vi "AlliGator Phasor Harmonic Manager.vi"() -> ()   [LabVIEW 2021, in "AlliGator Phasor Harmonics.lvlib"]
uses:
  AlliGator Phasor Harmonics.lvlib
  Phasor/Phasor Harmonic Frequency Information.ctl
  Image/Image Control Refnum.ctl
  Globals, Variables, Constants/AlliGator Refnums List.ctl
  Phasor Plot/AlliGator Phasor Harmonic Manager Actions.ctl
  Image/Image Display Event.ctl
  <vilib>/Utility/miscctls.llb/LVPoint32TypeDef.ctl
  Globals, Variables, Constants/AlliGator Variables List.ctl
  Variant/Variant to Data/Variant to String.vi
  Globals, Variables, Constants/AlliGator Globals, Variables & Constants.lvlib
  Action Engine/AlliGator Action Engine.lvlib
  Notebook/Notebook.lvlib
  Notebook/AlliGator Notebook.lvlib
  Variant/Variant to Data/Variant to Data.lvlib
  Phasor Plot/AlliGator Phasor Plot.lvlib
  Image/Image.lvlib
  Rich Text Box/Rich Text Box.lvlib
  Phasor/Phasor.lvlib
panel:
  in  "Phasor Harmonic List":i32[](listbox) caption="ROI List"
  out "Dataset File Paths":path[](array[path])
  out "Phasor Harmonic Descriptions":string[](array[string])
  out "Harmonic Frequencies Information":T1[](array[typedef]) {"Base Frequency" format="%#_5g"; "Phasor Frequency" format="%#_5g"}
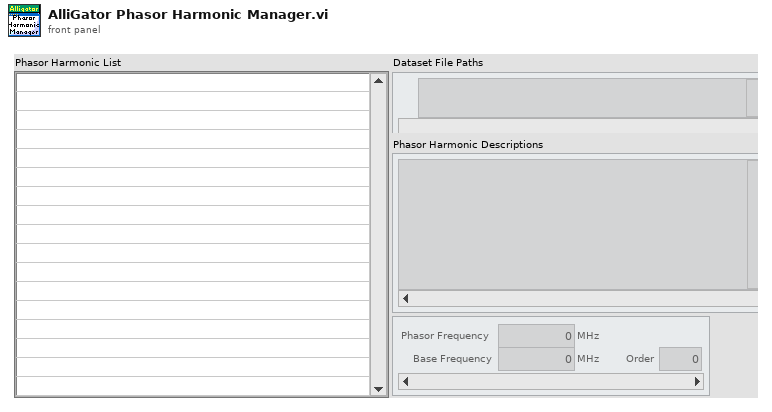
[diagram p1: front panel]
types:
  T1 = typedef "Phasor.lvlib/Phasor Harmonic Frequency Information.ctl" = cluster{"Phasor Frequency":dbl[unit], "Base Frequency":dbl[unit], "Order":u8}
  T2 = typedef "Image.lvlib/Image Control Refnum.ctl" = refnum<vi>
  T3 = typedef "AlliGator Globals, Variables & Constants.lvlib/AlliGator Refnums List.ctl" = enum16{"---------- AlliGator Controls ----------", "AlliGator Tab Control Refnum", "---------- AlliGator Indicators ----------", "Source Image Display Refnum", "Phasor Plot Display Refnum", "Decay Fit Parameter Map Refnum", "---------- AlliGator VIs ----------", "AlliGator Refnum", "AlliGator Settings Refnum", "AlliGator Launcher Refnum"}
  T4 = typedef "AlliGator Phasor Plot.lvlib/AlliGator Phasor Harmonic Manager Actions.ctl" = enum16{"Undefined", "Delete Current Harmonic", "Delete Multiple Harmonics", "Delete All Harmonics", "Swap Harmonics", "Insert Harmonics", "Rename Current Harmonic", "Store New Harmonic", "Store Multiple Harmonics", "Select Next Harmonic", "Select Previous Harmonic", "Update Phasor Harmonic Manager Window"}
  T5 = typedef "AlliGator Phasor Plot.lvlib/AlliGator Phasor Harmonic Manager Event Refnum.ctl" = refnum<user-event>
  T6 = typedef "Image.lvlib/Image Display Event.ctl" = cluster{"Item Tag":string, "Image Control Refnum":T2, "Coords":T7, "Item Path":string}
  T7 = typedef "LVPoint32TypeDef.ctl" = cluster{"Horizontal":i32, "Vertical":i32}
  T8 = typedef "AlliGator Globals, Variables & Constants.lvlib/AlliGator Variables List.ctl" = enum16{"---- GUI ----", "GUI:Initialization Status", "GUI:State Indicators Refnum", "GUI:Original AlliGator Menu Items", "GUI:Current Action Loop State", "GUI:Script in progress", "GUI:Playback", "GUI:Loop Playback", "GUI:Search ROI Used", "GUI:Search ROI", "Decay Graph Max Legend Size", "Intensity Graph Max Legend Size", "Decay Statistics Graph Max Legend Size", "Phasor Graph Max Legend Size", "Phasor Ratio Graph Max Legend Size", "Lifetime Graph Max Legend Size", "---- Files ----", "Files:Export Dataset Frames as Individual Files", "Files:Show Batch Export Help Balloons", "Files:Frames in Dataset", "Files:ptu File Frame Start Indices", "Files:Current Frame in Dataset", "Files:Current Frame Timestamp", "Files:Dataset Loaded", "Files:Dataset Metadata", "Files:Dataset Channel", "Files:Dataset Data Description", "Files:Background Dataset Metadata", "Files:Background Dataset Channel", "Files:Background Dataset Data Description", "Files:Background File Subtraction", "Files:Background File Path", "Files:Background File Pile-up Correction", "Files:Background File Pixel Well Capacity", "Files:Background File Scaling Factor", "Files:Current Dataset Load Settings", "Files:Dataset Path", "Files:ICCD-specific Information", "Files:Macrotime Gate Separation", "------ Python Plugins ------", "Python Plugins:Information", "Python Plugins:Python Session", "Python Plugins:Valid Python Session?", "---- Source Image ----", "Source Image:ROIs", "Source Image:Current ROI", "Source Image:ROI Event Refnum", "X_Source Image:Display Range", "X_Source Image:Palette Information", "X_Source Image:Type of Displayed Image", "X_Time Gate Slider", "Source Image:Palette List", "Source Image:Scale", "Source Image:ROI Overlay Color", "Source Image:Overlay to Erase", "Source Image:Is Displayed Image Accumulated", "Source Image:White Light Image Modified", "Source Image:Mask Image Modified", "---- Image Profile Window ----", "Image Profile:Window Event Refnum", "Image Profile:IntensityType", "Image Profile:Intensity Average Type", "Image Profile:Intensity-weighted SDV", "Image Profile:Box Profile Type", "Image Profile:Window Open", "Image Profile:Plotted Fit Parameter", "------ Phasor Graph -------", "Phasor Graph:Show Line", "---- Phasor Plot ---", "Phasor Plot:Parameters Changed", "Phasor Plot:FLI Dataset Modified since last Calculation", "Phasor Harmonics Data", "Selected Phasor Harmonics", "Phasor Harmonic Manager Event Refnum", "Phasor Plot:ROIs", "Phasor Plot:Current ROI", "Phasor Plot:ROI Event Refnum", "Phasor Plot:Image Reference Points", "Phasor Plot:Computed", "Phasor Plot:Palette Information", "Phasor Plot:Palette List", "Phasor Plot:Phasor Ratio Palette Information", "Phasor Plot:Phasor Ratio Palette List", "Phasor Plot:Image Scale", "Phasor Plot:Image Overlay to Erase", "Phasor Plot:Image Elements to Update", "Phasor Plot:Current Calculation Parameters", "Phasor Plot:Current Calibration Options", "Phasor Plot:Reset Cumulated Phasor Plot", "Phasor Plot:Reference 1", "Phasor Plot:Lifetime Reference 1", "Phasor Plot:Reference 1 Frequency", "Phasor Plot:Reference 2", "Phasor Plot:Lifetime Reference 2", "Phasor Plot:Reference 2 Frequency", "---- Decay Analysis ----", "Number of Selected Decays to Fit", "LS Fit Results", "LAR Fit Results", "BS Fit Results", "Last Decay Max - Min", "Best Fit Parameters", "Best Fit Parameter Names", "Actual Size X", "Actual Size Y", "Binning X", "Binning Y", "Actual # Gates", "Dataset Number", "Gates to...", "Gates Skipped", "Gates to keep", "Gate Step", "Gate Separation", "Reversed Gates", "Pile-up Correction", "Pixel Well Capacity", "Background Subtracted", "Background Subtraction Method", "Background Definition Range", "Background File (deprecated)", "Number of Dataset Accumulated", "Array of Accumulated Dataset Paths", "Do Averaged Datasets", "Destination File Path", "Process Plot Target", "Use 1/D as Phasor Frequency", "---- Decay Fit Parameter Map -----", "Decay Fit Parameter Map:Palette Information", "Decay Fit Parameter Map:Palette List", "Decay Fit Parameter Map:X Resolution", "Decay Fit Parameter Map:Y Resolution", "---- Parameter Map ----", "Parameter Map:Palette Information", "Parameter Map:Palette List", "------- Local Decay Window ---------", "Local Decay Graph Window:Event Refnum", "Local Decay Graph Window:Use normalized IRF for convolution", "----- Miscellaneous ----", "Misc:Skippable Dialog Windows Status"}
  T9 = cluster{"data name":string, "drag data":variant}[]
  T10 = typedef "AlliGator Action Engine.lvlib/AlliGator Q Element.ctl" = cluster{"AlliGator Q Event":T11, "Data":variant}
  T11 = typedef "AlliGator Action Engine.lvlib/AlliGator Q Event.ctl" = enum16{"---- Files ----", "Files:Set Batch Export Files To Save", "Files:Set Dataset Loading & Pre-processing Options", "Files:Check #Frames in Dataset", "Files:Increment Frame Index", "Files:Open Mask Image", "Files:Open White Light Image", "Files:Open Single Dataset", "Files:New Folder of Folders Selected", "Files:Load File (all Types)_Scriptable", "Files:Move Flattened Series to Folders Series", "Files:Select Folder", "Files:Load FLI Dataset", "Files:Load Swiss SPAD 1 Dataset", "Files:Load Swiss SPAD 2 Dataset", "Files:Load .sdt FLI Dataset", "Files:Load .ptu FLI Dataset", "Files:Load .bin FLI Dataset", "Files:Load Single Gate Image Folder", "Files:Load I/m/phi Dataset (deprecated)", "Files:Load Single Image", "Files:Subtract Background File", "Files:Export FLI Dataset", "Files:Load HDF5 FLI Dataset", "Files:Set Destination File Path", "Files:Save Mask Image", "Files:Batch Conversion", "Files:New Folder Selected", "Files:Close FLI Dataset", "Files:Close FLI Dataset Series", "Files:Close White Light Image", "Files:Close Mask Image", "---- FLI Dataset ----", "FLI Dataset:Channel Arithmetic", "FLI Dataset:Export Average Lifetime Map as ASCII", "FLI Dataset:Export User-Defined Quantity Map as ASCII", "FLI Dataset:Python Function FLI Dataset Event", "FLI Dataset:ROI Analysis", "FLI Dataset:Tilted Logistic Square Gated IRF Characteristics Map", "FLI Dataset:Logistic Square Gated IRF Characteristics Map", "FLI Dataset:Square Gated IRF Characteristics Map", "FLI Dataset:Multi-ROI Single-Pixel Phasor Analysis", "FLI Dataset:Multi-ROI Single-Pixel NLSF Analysis", "FLI Dataset:All ROIs IRF Extraction", "FLI Dataset:All ROIs Decay Fit Non-Interactive (Fast + Individual IRF)", "FLI Dataset:All ROIs Phasor Analysis", "FLI Dataset:All ROIs Decay Fit", "FLI Dataset:Fluorescence Decay Statistics", "FLI Dataset:Update Decay Statistics Graph", "FLI Dataset:Get Decay from ROI", "FLI Dataset:All ROIs Average Lifetimes", "FLI Dataset:Save/Load Local IRFs", "FLI Dataset:Clear Local IRFs", "---- FLI Dataset Series ----", "FLI Dataset Series:Sum All Datasets in Series", "FLI Dataset Series:Add Dataset to Accumulated Dataset", "FLI Dataset Series:Display Accumulated Dataset", "FLI Dataset Series:Clear Dataset Series Sum", "FLI Dataset Series:Time-Series Analysis (NLSF)", "FLI Dataset Series:Time-Series Analysis (Phasor)", "---- Image ----", "Image:Update Image Profile Plots", "Image:Image Histogram Cursor Move", "Image:Image Histogram", "Image:Image Contrast", "Image:Set Image Histogram Cursor Move Flag", "Image:Clear Image Overlay", "Image:Use ROI as Search Area", "Image:Set ROI Diameter", "Image:Save Image Data as TIFF", "Image:Save Displayed Image with Overlay", "Image:Save Image Overlay Only", "Image:Save Image as Hot Pixel Mask", "Image:Change Source Image Color Palette", "Image:Copy Image to Clipboard", "Image:Source Image ROI Selection", "Image:Delete All ROIs", "Image:Delete All Unselected ROIs", "Image:Delete ROI", "Image:Merge All ROIs", "Image:Store ROI", "Image:Source Image ROI Storage", "Image:Export ROI Description to Notebook", "Image:Save ROI", "Image:Load ROI", "Image:Paste ROI Definition", "Image:Clear ROI", "Image:Identify ROIs in Mask Image", "Image:Create Complementary ROI", "Image:Create Contour ROI", "Image:Create ROI(s) from Pixels with Peak above Min_Scriptable", "Image:Create ROI(s) from Pixels with Intensity above Min_Scriptable", "Image:Compute ROI Statistics", "Image:Delete ROI(s) based on ROI Characteristics", "Image:Create ROI Grid", "Image:ROI to Individual Pixel ROIs", "Image:Python Function Source Image Event", "Image:Show Phasor Calibration Map ROI Centers", "Image:Convert ROI to Mask Image", "Image:Mouse Move", "Image:Mouse Up", "Image:Set Source Image Mouse Move Flag", "Image:Add Scale Bar Overlay", "Image:Delete Existing ROIs Option", "Image:Overlay ROI Median", "Image:Check Current ROI", "---- Decay ----", "Decay:Clear IRF/Reference Plot", "Decay:Add Decay to Graph", "Decay:Smoothen Plot", "Decay:Smoothen Plot Tail", "Decay:Average Selected Plots", "Decay:Extract IRF", "Decay:Optimal IRF Extraction", "Decay:Threshold IRF", "Decay:Fit to Model IRF", "Decay:Fit IRF to Square Gate", "Decay:Fit IRF to Logistic Square Gate", "Decay:Fit IRF to Tilted Logistic Square Gate", "Decay:Create Bounding Cursors Set", "Decay:Export Bounding Cursors Definition to Notebook", "Decay:Denoise Plot", "Decay:Compute Cumulative Function", "Decay:Use as Reference Decay", "Decay:Show Reference Decay/IRF", "Decay:Extrapolate Decay", "Decay:Create Head & Tail Bounding Cursors", "Decay:Store Cursor-defined Head & Tail Fractions", "Decay:Rebin Plot", "Decay:1-Normalize Decay", "Decay:[0-1]-Normalize Plot", "Decay:Straighten Decay", "Decay:Shift Decay", "Decay:Fold Decay", "Decay:Fit Decay", "Decay:Global Fit of Selected Decays", "Decay:Post Global Fit Script", "Decay:Add Global Fit Parameters to Graph", "Decay:Add Decay Parameter(s) to Plot (Graph)", "Decay:Export Decay to Phasor Graph", "Decay:Plot Decay Shifts", "Decay:Compute Average Lifetime", "Decay:Plot Convolution", "Decay:Graph Tip Strip Update", "---- Decay Statistics ----", "Decay Statistics:Tip Strip Update", "---- Intensity Time Trace ----", "Intensity Time Trace:Use File Timestamp", "Intensity Time Trace:Load Intensity Corrections File", "Intensity Time Trace:Clear Intensity Corrections File", "Intensity Time Trace:Tip Strip Update", "---- Phasor Plot ----", "Phasor Plot:Build Phasor Plot", "Phasor Plot:Change Phasor Plot Color Palette", "Phasor Plot:Adjust Phasor Plot Display Range", "Phasor Plot:Highlight Image ROI in Phasor Plot", "Phasor Plot:Save Phasor Plot Image with Overlay", "Phasor Plot:Export Complex Phasor Map", "Phasor Plot:Export Phasor Ratio Map", "Phasor Plot:Export Average Lifetime Map", "Phasor Plot:Compute Phase Lifetime Histogram", "Phasor Plot:Compute Phasor Ratio Histogram", "Phasor Plot:Compute Phase Lifetime vs Intensity Scatter Plot", "Phasor Plot:Weber 2-Component Decomposition", "Phasor Plot:Update Phasor Color Map Vertices", "Phasor Plot:Clear Phasor Overlay", "Phasor Plot:Use Segment Extremities as References", "Phasor Plot:Use UC/Segment Intersections as References", "Phasor Plot:Use UC/Principal Axis Intersections as References", "Phasor Plot:Use UC/Linear Fit Intersections as References", "Phasor Plot:Update Phasor Plot Reference", "Phasor Plot:Show Local Phasor Info in Phasor Plot", "Phasor Plot:Update Phasor Plot State", "Phasor Plot:Phasor Plot ROI Storage", "Phasor Plot:Phasor Plot ROI Selection", "Phasor Plot:Python Function Phasor Plot Event", "Phasor Plot:Overlay Phasor ROI, Ratio or Map in Source Image", "Phasor Plot:Compute Decay of Selected Phasors", "Phasor Plot:Phasor at Image Pixel", "Phasor Plot:Mouse Move", "Phasor Plot:Mouse Up", "Phasor Plot:Display Range Mouse Move", "Phasor Plot:Set Mouse Move Flag", "---- Phasor Graph ----", "Phasor Graph:Calibrated Phasor Map Series", "Phasor Graph:Whole Image Phasor Scatter Plot (deprecated)", "Phasor Graph:Get Phasor Value", "Phasor Graph:Create New Phasor Plot Dialog", "Phasor Graph:Update Last Phasor Value", "Phasor Graph:Update Phasor (m, phi)", "Phasor Graph:Remove Single Phasor from Plot", "Phasor Graph:Add Single Phasor to Plot", "Phasor Graph:Remove Phasor Plot", "Phasor Graph:Remove Selected Phasor Plots", "Phasor Graph:Clear Phasor Data", "Phasor Graph:Clear Phasor Graph", "Phasor Graph:Cursor Move", "Phasor Graph:Draw Cursor Connecting Line", "Phasor Graph:Clear Cursor Connecting Line", "Phasor Graph:Find UC Intersection", "Phasor Graph:Use UC/Cursor-Defined Line Intersections", "Phasor Graph:Use Selected Plots Fitted Line/UC Intersections", "Phasor Graph:Use Selected Plots Principal Axis/UC Intersections", "Phasor Graph:Show Single Phasor", "Phasor Graph:Save Single Phasor Plot", "Phasor Graph:Save All Phasor Plots", "Phasor Graph:Load Phasor Plot(s)", "Phasor Graph:Phasor Multiplication", "Phasor Graph:Compute Average Phasor", "Phasor Graph:Compute Multiple Average Phasors (Selected Plots)", "Phasor Graph:Export Single Phasor Plot Phase Lifetimes", "Phasor Graph:Phase Lifetime Trajectory (deprecated)", "Phasor Graph:Phase Lifetime vs Intensity Scatter Plot (deprecated)", "Phasor Graph:Parameter 2 vs Parameter 1 Scatter Plot", "Phasor Graph:Use Cursor n Location", "Phasor Graph:Set Reference n to Current Phase Lifetime Value", "Phasor Graph:Set Reference n to Lifetime Value", "Phasor Graph:Set Cursor n Location", "Phasor Graph:Save Phasor Graph Image", "Phasor Graph:Update SEPL Plot", "Phasor Graph:Export Single Phasor Plot Data", "Phasor Graph:Export Selected Phasor Plots Data", "Phasor Graph:Python Function Phasor Graph Event", "Phasor Graph:Tip Strip Update", "---- Calibration ----", "Calibration:Set Calibration Type", "Calibration:Load/Save Phasor Calibration", "Calibration:Load/Save Phasor Calibration Series", "Calibration:Load/Save Phasor Calibration Map", "Calibration:Use as Calibration", "Calibration:Compute Optimal Calibration from Phasor References", "Calibration:Clear Phasor Calibration", "Calibration:Single Phasor Calibration Information", "Calibration:Use as Calibration Series", "Calibration:Use as Calibration Map", "Calibration:Clear Calibration Series", "Calibration:Phasor Calibration Series Information", "Calibration:Clear Calibration Map", "Calibration:Phasor Calibration Map Information", "Calibration:Apply Phasor Calibration", "Calibration:Update Single Plot Calibration", "Calibration:Update Multiple Plots Calibration", "Calibration:Clear Single Plot Calibration", "Calibration:Clear All Plots Calibrations", "Calibration:Clear Plot(s) Calibration(s)?", "Calibration:Phasor Calibration Maps (# Gates Series)", "---- Phasor Ratio ----", "Phasor Ratio:Clear Reference n", "Phasor Ratio:Toggle Selected Plot(s)  Lock to Reference 1", "Phasor Ratio:Use as Reference n", "Phasor Ratio:Send Reference n to Notebook", "Phasor Ratio:Toggle Selected Plot(s)  Lock to Reference 2", "Phasor Ratio:Compute Phasor Ratio at Mouse Location", "Phasor Ratio:Compute Phasor Plot's Average Phasor Ratio", "Phasor Ratio:Compute Time-Series Phasor Ratios", "Phasor Ratio:Fit Line to Phasor Ratio Plot", "Phasor Ratio:Save References", "Phasor Ratio:Load References", "Phasor Ratio:Update Phasor Reference 1", "Phasor Ratio:Update Phasor Reference 2", "Phasor Ratio:Move Cursor n to Reference n", "Phasor Ratio:Use as Phasor Reference 1 Lifetime", "Phasor Ratio:Use as Phasor Reference 2 Lifetime", "Phasor Ratio:Export Phasor Ratio Map as ASCII", "Phasor Ratio:Tip Strip Update", "---- Lifetime & Other Parameters Graph ----", "Lifetime:Power Law from Intensity Distribution", "---- Decay Fit Parameter Map ----", "Decay Fit Parameter Map:Export ROI NLSF Data as ASCII", "Decay Fit Parameter Map:Set Decay Fit Parameter Map Selection", "Decay Fit Parameter Map:Build Decay Fit Parameter Map", "Decay Fit Parameter Map:Change Decay Fit Parameter Map Color Palette", "Decay Fit Parameter Map:Export Decay Fit Parameter Map Data as ASCII", "Decay Fit Parameter Map:Export All Decay Fit Parameter Maps Data as ASCII", "Decay Fit Parameter Map:Selected Parameter Scatterplot", "Decay Fit Parameter Map:Parameter 2 vs Parameter 1 Scatterplot", "Decay Fit Parameter Map:Save Decay Fit Parameter Map Image", "Decay Fit Parameter Map:Save-Load IRFs & Fit Data", "Decay Fit Parameter Map:Update Local Decay Plots", "Decay Fit Parameter Map:Python Function Decay Fit Parameters Map Event", "Decay Fit Parameter Map:Overlay Decay Fit Parameter Map in Source Image", "Decay Fit Parameter Map:Selected Parameter vs Intensity Scatterplot", "Decay Fit Parameter Map:Mouse Up", "Decay Fit Parameter Map:Display Range Mouse Move", "Decay Fit Parameter Map:Change Map Resolution", "---- Parameter Map ----", "Parameter Map:Export ROI Parameters Data as ASCII", "Parameter Map:Delete Parameter Map Set", "Parameter Map:Update Parameter List", "Parameter Map:Build Parameter Map", "Parameter Map:Change Parameter Map Color Palette", "Parameter Map:Export Parameter Map Data as ASCII", "Parameter Map:Export All Parameter Maps Data as ASCII", "Parameter Map:Selected Parameter Scatterplot", "Parameter Map:Parameter 2 vs Parameter 1 Scatterplot", "Parameter Map:Selected Parameter vs Intensity Scatterplot", "Parameter Map:Save Parameter Map Image", "Parameter Map:Save-Load IRFs & Parameter Maps (TODO)", "Parameter Map:Set Parameter Map Selection", "Parameter Map:Python Function Parameter Map Event", "Parameter Map:Overlay Parameter Map in Source Image", "Parameter Map:Update Local Decay Plots", "Parameter Map:Mouse Up", "Parameter Map:Display Range Mouse Move", "---- Generic Graph ----", "Generic Graph:Generic XY Graph Event", "Generic Graph:Python Function XY Graph Event", "Generic Graph:New Plot", "Generic Graph:Save Plot", "Generic Graph:XY Plot Histogram", "Generic Graph:Set XY Graph Plot Name", "Generic Graph:Set Last Cursor Style", "Generic Graph:Tip Strip Update", "---- GUI ----", "GUI:Start Script", "GUI:Type of Displayed Image Changed", "GUI:Gate Image Slide Changed", "GUI:Show Busy Icon", "GUI:Show Busy Icon & Abort Button", "GUI:Hide Busy Icon", "GUI:Hide Busy Icon & Abort Button", "GUI:Abort", "GUI:End Script", "GUI:Start Timing", "GUI:End Timing", "GUI:Set State Indicator", "GUI:Send Parameters JSON Strings to Clipboard", "GUI:Set Gate Step", "GUI:Idle", "GUI:Initialization", "GUI:Quit", "GUI:Increment Dataset Index", "GUI:Set Dataset Index to -1", "GUI:Time Series Slider Moved", "GUI:Time Series Slider Changed", "GUI:Toggle Playback or Loop", "GUI:Playback Script", "GUI:Set Phasor Frequency", "GUI:Open Window", "GUI:Start Test Script", "GUI:End Test Script", "DEBUG"}
  T12 = typedef "Rich Text Box.lvlib/Text Formatting.ctl" = cluster{"Font":string, "Text Color":T13, "Text Background Color":T13, "Text Style":enum16{"Regular", "Bold", "Italic", "Underline", "Strikeout"}, "Font Size (Points)":dbl, "Text Alignment":i32}
  T13 = typedef "Rich Text Box.lvlib/Text Colors.ctl" = enum16{"Unchanged", "Black", "Blue", "Brown", "Gray", "Green", "Orange", "Pink", "Red", "White"}
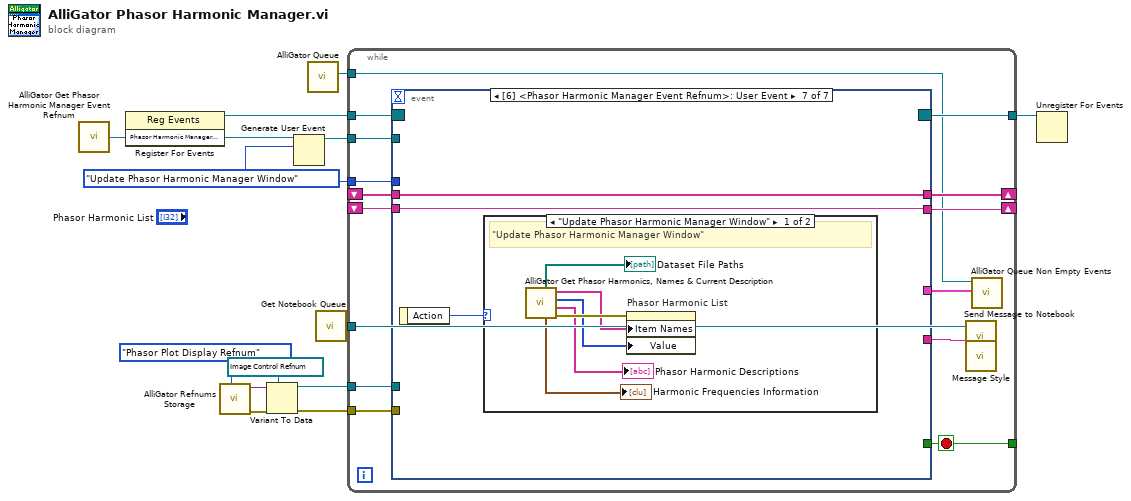
[diagram p0: block diagram]
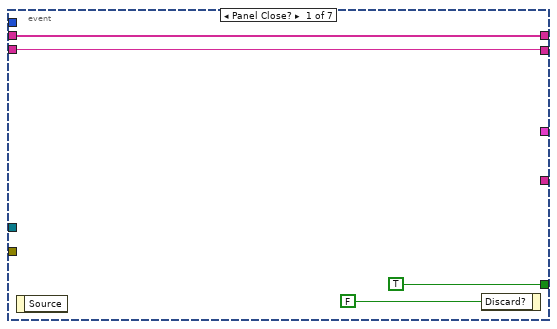
[diagram p2: hidden frame]
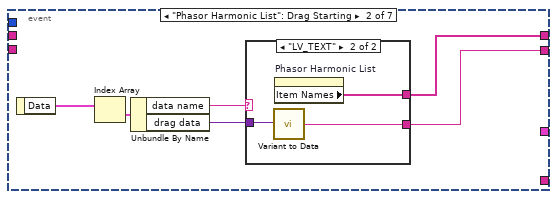
[diagram p3: hidden frame]
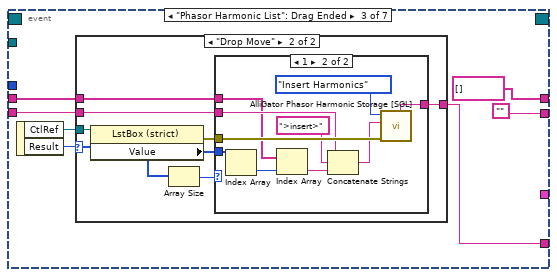
[diagram p5: hidden frame]
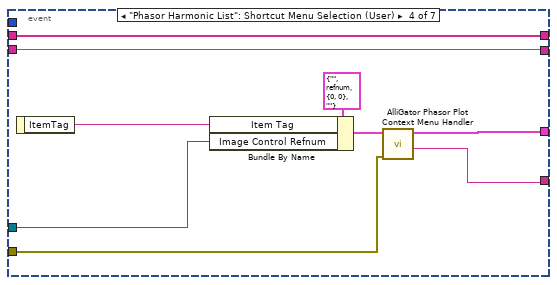
[diagram p8: hidden frame]
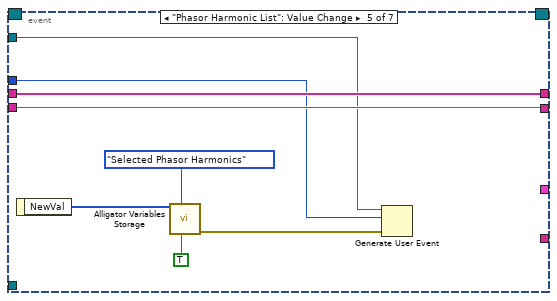
[diagram p9: hidden frame]
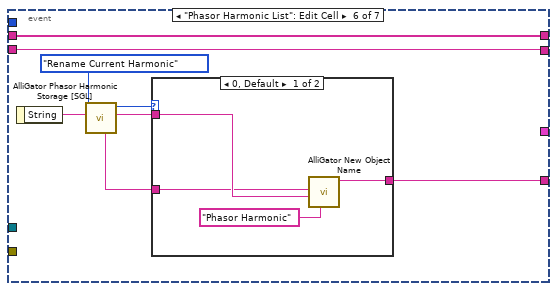
[diagram p10: hidden frame]
diagram:
  w7 = AlliGator_Phasor_Harmonic_Manager_Actions."Update Phasor Harmonic Manager Window" ("event data")
  n1 = call "AlliGator Get Phasor Harmonic Manager Event Refnum.vi"() -> ("Phasor Harmonic Manager Event Refnum"=w9:T5)
  n2 = register-events(w9) -> (reference out=w13:refnum<event-registration>)  [unwired: 2 in, 1 out]
  n3 = call "AlliGator Refnums Storage.vi"("AlliGator Refnum List"=AlliGator_Refnums_List."Phasor Plot Display Refnum") -> ("Error Out"=w6:errorcluster, "Data out"=w5:variant)  [unwired: 9 in]
  n4 = Variant To Data(error in=w6, type=T2 refnum ("Image Control Refnum"), Variant=w5) -> (data=w1:T2, error out=w3:errorcluster)
  n5 = Generate User Event(user event=w9, event data cluster=w7) -> (user event out=w8:T5)  [unwired: 2 in, 1 out]
  n6 = call "AlliGator Queue.vi"() -> ("AlliGator Q"=w11:refnum<queue>)  [unwired: 8 in, 1 out]
  n7 = call "Get Notebook Queue.vi"() -> ("Notebook Queue"=w10:refnum<queue>)  [unwired: 9 in]
  n8 = while {
    tunnel: w13 -> [w29]
    tunnel: [w28] -> w12
    tunnel: w11 -> [w20]
    tunnel: w10 -> [w14]
    shift-right: [w27] -> _
    shift-left: _ -> [w26]
    shift-right: [w25] -> _
    shift-left: _ -> [w24]
    tunnel: w8 -> [w23]
    tunnel: w7 -> [w22]
    tunnel: [w21] -> _
    tunnel: w3 -> [w18]
    tunnel: w1 -> [w17]
    stop <- w21 stop-if-true
    n9 = event shown="[6] <Phasor Harmonic Manager Event Refnum>: User Event" {
      selector: w29 -> [_ _ _ _ _ _ _]
      dyn-events: [_ _ _ _ _ _ _] -> w28
      timeout: _ -> [_ _ _ _ _ _ _]
      tunnel: [TRUE _ _ _ _ _ _] -> w21
      tunnel: [w31 w36 "" w75 w82 w91 w98] -> w27
      tunnel: w26 -> [w31 _ w47 w75 w82 w91 w98]
      tunnel: [w30 w34 string[] [] ("Item Names") w74 w81 w90 w97] -> w25
      tunnel: w24 -> [w30 _ w45 w74 w81 w90 w97]
      tunnel: w23 -> [_ _ _ _ w78 _ _]
      tunnel: w22 -> [_ _ _ _ w77 _ _]
      tunnel: [_ _ _ w71 _ _ _] -> w19
      tunnel: w18 -> [_ _ _ w69 _ _ _]
      tunnel: w17 -> [_ _ _ w68 _ _ _]
      tunnel: [_ _ w43 w67 _ w84 _] -> w15
      event Panel Close? {
        n10 = event-data() -> ()  [unwired: 1 in, 1 out]
        n11 = event-data("Discard?"=FALSE) -> ()  [unwired: 1 in, 1 out]
      }
      event "Phasor Harmonic List": Drag Starting {
        n12 = event-data() -> ("Data"=w39:T9)  [unwired: 1 in]
        n13 = Index Array(array=w39) -> (element=w38:cluster{"data name":string, "drag data":variant})  [unwired: 1 in]
        n14 = Unbundle By Name(w38) -> ("data name"=w37:string, "drag data"=w35:variant)
        n15 = case shown="\"LV_TEXT\"" w37 {
          tunnel: [_ w41] -> w36
          tunnel: w35 -> [_ w42]
          tunnel: [_ w40] -> w34
          frame "False", Default {
          }
          frame "LV_TEXT" {
            n16 = call-poly "Variant to Data.vi"("Variant"=w42) -> ("String"=w41:string)  [unwired: 8 in]
            n17 = property on="Phasor Harmonic List" class="LstBox (strict)"() -> ("Item Names"=w40:string[])  [unwired: 2 in, 2 out]
          }
        }
      }
      event "Phasor Harmonic List": Drag Ended {
        n18 = event-data() -> ("CtlRef"=w49:refnum<vi>, "Result"=w48:enum16{"Drop Cancel", "Drop Move", "Drop Copy"})  [unwired: 1 in]
        n19 = case shown="\"Drop Move\"" w48 {
          tunnel: w49 -> [_ w56]
          tunnel: w47 -> [_ w54]
          tunnel: w45 -> [_ w53]
          tunnel: [_ w50] -> w43
          frame "Drop Cancel", Default {
          }
          frame "Drop Move" {
            n20 = property class="LstBox (strict)"(reference=w56) -> (error out=w55:errorcluster, "Value"=w51:i32[])  [unwired: 1 in, 1 out]
            n21 = Array Size(array=w51) -> (size(s)=w52:i32)
            n22 = case shown="1" w52 {
              tunnel: w55 -> [_ w66]
              tunnel: w54 -> [_ w62]
              tunnel: w53 -> [_ w61]
              tunnel: w51 -> [_ w59]
              tunnel: [_ w57] -> w50
              frame 0, Default {
              }
              frame 1 {
                n23 = Index Array(array=w59) -> (element=w58:i32)  [unwired: 1 in]
                n24 = Index Array(array=w61, index=w58) -> (element=w65:string)
                n25 = Concatenate Strings(w62, ">insert>" ("string"), w65) -> (w64:string)
                n26 = call "AlliGator Phasor Harmonic Storage [SGL].vi"("Error In"=w66, "Default Name (\"Phasor Harmonic\")"=w64, "Action"=AlliGator_Phasor_Harmonic_Manager_Actions."Insert Harmonics") -> ("Message"=w57:string)  [unwired: 3 in, 5 out]
              }
            }
          }
        }
      }
      event "Phasor Harmonic List": Shortcut Menu Selection (User) {
        n27 = event-data() -> ("ItemTag"=w72:string)  [unwired: 1 in]
        n28 = Bundle By Name(cluster=T6 {"Item Tag"="", "Image Control Refnum"=refnum, "Coords"={"Horizontal"=0, "Vertical"=0}, "Item Path"=""} ("Image Event Data"), "Item Tag"=w72, "Image Control Refnum"=w68) -> (w70:T6)
        n29 = call "AlliGator Phasor Plot Context Menu Handler.vi"("Error In"=w69, "Image Event"=w70) -> ("Message"=w67:string, "AlliGator Actions"=w71:T10[])  [unwired: 7 in, 1 out]
      }
      event "Phasor Harmonic List": Value Change {
        n30 = event-data() -> ("NewVal"=w83:i32[])  [unwired: 1 in]
        n31 = call "Alligator Variables Storage.vi"("Get(F)/Set"=TRUE, "AlliGator Variable"=AlliGator_Variables_List."Selected Phasor Harmonics" ("Alligator Variable"), "Data in"=w83) -> ("Error Out"=w76:errorcluster)  [unwired: 6 in, 2 out]
        n32 = Generate User Event(user event=w78, event data cluster=w77, error in=w76) -> ()  [unwired: 1 in, 2 out]
      }
      event "Phasor Harmonic List": Edit Cell {
        n33 = event-data() -> ("String"=w89:string)  [unwired: 1 in]
        n34 = call "AlliGator Phasor Harmonic Storage [SGL].vi"("Default Name (\"Phasor Harmonic\")"=w89, "Action"=AlliGator_Phasor_Harmonic_Manager_Actions."Rename Current Harmonic") -> ("Current Phasor Harmonic Name"=w87:string, "Current Phasor Harmonic Index"=w85:i32, "Old Phasor Harmonic Name"=w86:string)  [unwired: 4 in, 3 out]
        n35 = case shown="0, Default" w85 {
          tunnel: w87 -> [w94 _]
          tunnel: w86 -> [w93 _]
          tunnel: [w92 _] -> w84
          frame 0, Default {
            n36 = call "AlliGator New Object Name.vi"("Object String ('ROI')"="Phasor Harmonic", "Modified Object Name"=w94, "Original Object Name"=w93) -> ("Message"=w92:string)  [unwired: 7 in, 1 out]
          }
          frame -1 {
          }
        }
      }
      event User Event {
        n37 = event-data() -> ("Action"=w96:T4)  [unwired: 1 in]
        n38 = case shown="\"Update Phasor Harmonic Manager Window\"" w96 {
          frame "Update Phasor Harmonic Manager Window" {
            # "\"Update Phasor Harmonic Manager Window\""
            n39 = call "AlliGator Get Phasor Harmonics, Names & Current Description.vi"() -> ("Error Out"=w104:errorcluster, "Current Phasor Harmonic Parameter Strings"=→"Phasor Harmonic Descriptions":string[], "Current Phasor Harmonics"=w100:i32[], "Phasor Harmonics Names"=w103:string[], "Phasor Harmonic Fequency Informations"=→"Harmonic Frequencies Information":T1[], "Dataset File Paths"=→"Dataset File Paths":path[])  [unwired: 6 in]
            n40 = property on="Phasor Harmonic List" class="LstBox (strict)"(error in=w104, "Item Names"=w103, "Value"=w100) -> ()  [unwired: 1 in, 2 out]
          }
          frame Default {
          }
        }
      }
    }
    n41 = call "Message Style.vi"() -> ("Message Formatting"=w16:T12)
    n42 = call "Send Message to Notebook.vi"("Text Formatting"=w16, "Message"=w15, "Notebook Queue"=w14) -> ()  [unwired: 5 in, 2 out]
    n43 = call "AlliGator Queue Non Empty Events.vi"("Actions"=w19, "AlliGator Q"=w20) -> ()  [unwired: 9 in, 1 out]
  }
  n44 = Unregister For Events(event registration refnum=w12) -> ()  [unwired: 1 in, 1 out]
